vi "SP Append Measured Waveform.vi"(0 "Waveforms in":waveform(dbl)[](array[waveform]), 1 "Attribute Name (NI_ChannelName)":string="NI_ChannelName", 2 "CH Controls":T1[](array[typedef]) {"Measure" items=["S11", "S21", "S12", "S22"]; "Reference" format="%#.2g"; "Display Data" items=["Data", "Memory", "Data/Memory"]; "Format" items=["Log Mag", "Phase", "Expanded Phase", "Delay", "Smith", "Polar", "Lin Mag", "SWR", "Loss", "Real", "Imaginary"]; "Scale" min=0.001 step=1.0 format="%#.2g"; "Position" min=0.0 max=10.0}, 5 "Measured Data":cdb[](array[numeric]), 7 "All Measured Data":cdb[][](array[numeric]), 9 "Current Index":i32, 11 "error in (no error)":errorcluster, 12 "Number of Parameters Measured":i32, 14 "Measured Parameter":T4={"Stimulus Port"=1, "Response Port"=1} {"Stimulus Port" min=1 step=1; "Response Port" min=1 step=1}) -> (4 "Waveforms out":waveform(dbl)[](array[waveform]), 6 "Memory Exists?":bool, 10 "Stored Data":cdb[](array[numeric]), 15 "error out":errorcluster)   [LabVIEW 2011]
uses:
  TypeDefs/SP Parameter.ctl
  TypeDefs/SP Display Trace Controls.ctl
  TypeDefs/SP Display Format.ctl
  TypeDefs/SP Display Data.ctl
  TypeDefs/SP Format.ctl
  TypeDefs/SP Channel Type.ctl
panel:
  # "Div"
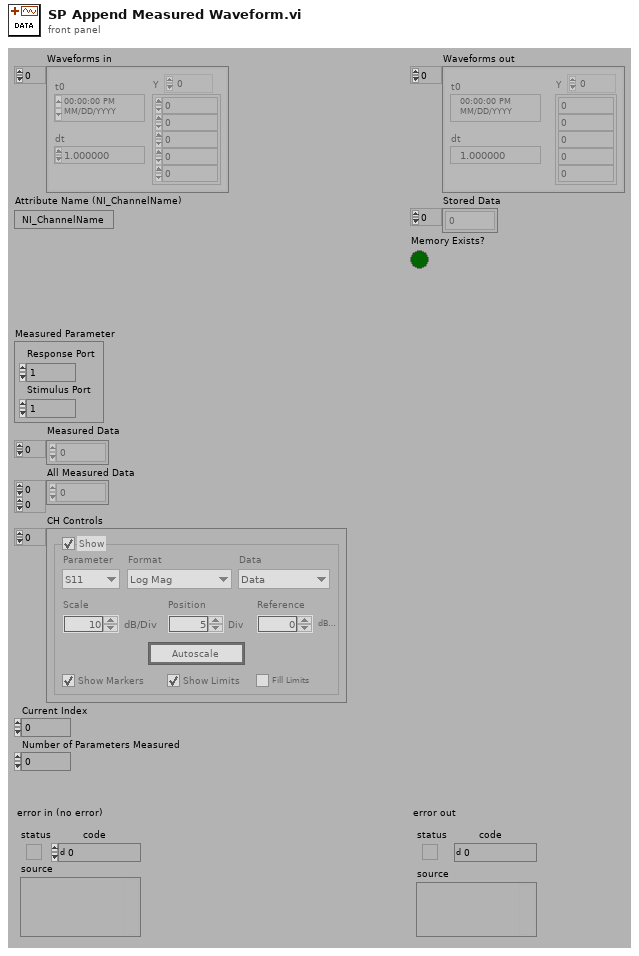
[diagram p1: front panel]
types:
  T1 = typedef "SP Display Trace Controls.ctl" = cluster{"Trace On":bool, "Measure":i32, "Format":T2, "Autoscale":bool, "Reference":dbl, "\nRefUnit":string, "Position":dbl, "Scale":dbl, "ScaleUnit":string, "LimitOn":bool, "LimitFill":bool, "Display Data":T3, "Show Markers":bool, "SXX":string}
  T2 = typedef "SP Display Format.ctl" = i32
  T3 = typedef "SP Display Data.ctl" = u16
  T4 = typedef "SP Parameter.ctl" = cluster{"Stimulus Port":i8, "Response Port":i8}
  T5 = typedef "SP Channel Type.ctl" = enum16{"Frequency", "Data", "Limit", "Adapter", "Memory", "Value", "Value Limit"}
  T6 = typedef "SP Format.ctl" = enum16{"Log Mag", "Lin Mag", "SWR", "Phase", "Expanded Phase", "Delay", "Insertion Loss", "Isolation", "Return Loss"}
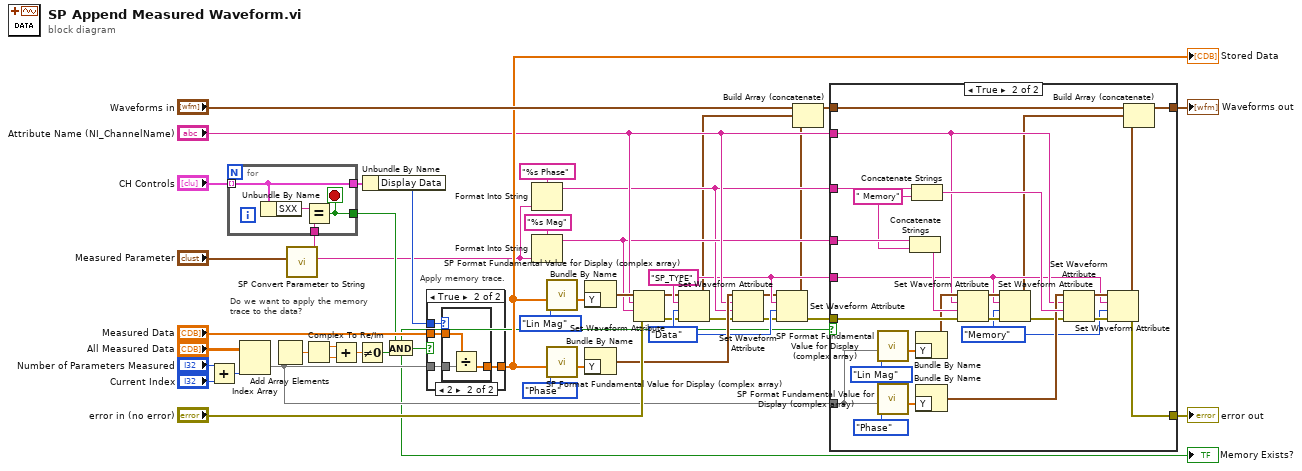
[diagram p0: block diagram]
diagram:
  w10 = "SP_TYPE" ("string")
  w11 = SP_Channel_Type."Data" ("Channel Type")
  # "Apply memory trace."
  # "Do we want to apply the memory\ntrace to the data?"
  n1 = Add(x="Number of Parameters Measured", y="Current Index") -> (x+y=w28:i32)
  n2 = Index Array(array="All Measured Data", index (col)=w28) -> (element=w14:cdb[])  [unwired: 1 in]
  n3 = Add Array Elements(numeric array=w14) -> (sum=w26:cdb)
  n4 = call "SP Convert Parameter to String.vi"("Parameter"="Measured Parameter") -> ("Parameter String"=w12:string)  [unwired: 10 out]
  n5 = for {
    tunnel: "CH Controls" -> [w48] mode=indexing
    tunnel: w12 -> [w49]
    tunnel: [w47] -> w21
    tunnel: [w48] -> w41
    stop <- w47 stop-if-true
    n6 = Unbundle By Name(w48) -> ("SXX"=w46:string)
    n7 = Equal?(x=w46, y=w49) -> (x = y?=w47:bool)
  }
  n8 = Complex To Re/Im(x + iy=w26) -> (x=w25:dbl, y=w24:dbl)
  n9 = Add(x=w25, y=w24) -> (x+y=w23:dbl)
  n10 = Not Equal To 0?(x=w23) -> (x != 0?=w1:bool)
  "Memory Exists?" <- w1
  n11 = Unbundle By Name(w41) -> ("Display Data"=w22:T3)
  n12 = And(x=w21, y=w1) -> (x .and. y?=w27:bool)
  n13 = case shown="True" w27 {
    tunnel: "Measured Data" -> [w50 w54]
    tunnel: [w50 w53] -> w29
    tunnel: w14 -> [_ w52]
    tunnel: w22 -> [_ w51]
    frame False {
    }
    frame True {
      n14 = case shown="2" w51 {
        tunnel: w54 -> [w55 w58]
        tunnel: [w55 w57] -> w53
        tunnel: w52 -> [_ w56]
        frame Default {
        }
        frame 2 {
          n15 = Divide(x=w58, y=w56) -> (x/y=w57:cdb[])
        }
      }
    }
  }
  "Stored Data" <- w29
  n16 = Format Into String(format string="%s Phase", w12) -> (resulting string=w17:string)  [unwired: 2 in, 1 out]
  n17 = Format Into String(format string="%s Mag", w12) -> (resulting string=w18:string)  [unwired: 2 in, 1 out]
  n18 = call "SP Format Fundamental Value for Display (complex array).vi"("Sxx Measured Format"=SP_Format."Lin Mag" ("Sxx Measure Format"), "Fundamental Values"=w29) -> ("Formatted Values"=w33:dbl[])  [unwired: 1 in, 8 out]
  n19 = call "SP Format Fundamental Value for Display (complex array).vi"("Sxx Measured Format"=SP_Format."Phase" ("Sxx Measure Format"), "Fundamental Values"=w29) -> ("Formatted Values"=w32:dbl[])  [unwired: 1 in, 8 out]
  n20 = Bundle By Name("Y"=w33) -> (w37:waveform(dbl))  [unwired: 1 out]
  n21 = Bundle By Name("Y"=w32) -> (w34:waveform(dbl))  [unwired: 1 out]
  n22 = Set Waveform Attribute(4:"error in (no error)", 5:w18, 6:"Attribute Name (NI_ChannelName)", 7:w37) -> (0:w4:errorcluster, 3:w5:waveform(dbl))  [unwired: 1 out]
  n23 = Set Waveform Attribute(4:w4, 5:w11, 6:w10, 7:w5) -> (0:w8:errorcluster, 3:w7:waveform(dbl))  [unwired: 1 out]
  n24 = Set Waveform Attribute(4:w8, 5:w17, 6:"Attribute Name (NI_ChannelName)", 7:w34) -> (0:w2:errorcluster, 3:w3:waveform(dbl))  [unwired: 1 out]
  n25 = Set Waveform Attribute(4:w2, 5:w11, 6:w10, 7:w3) -> (0:w9:errorcluster, 3:w6:waveform(dbl))  [unwired: 1 out]
  n26 = Build Array (concatenate)("Waveforms in", w7, w6) -> (w16:waveform(dbl)[])
  n27 = case shown="True" w1 {
    tunnel: w9 -> [w59 w86]
    tunnel: [w59 w63] -> w20
    tunnel: "Attribute Name (NI_ChannelName)" -> [_ w74]
    tunnel: w18 -> [_ w73]
    tunnel: w17 -> [_ w71]
    tunnel: w16 -> [w60 w83]
    tunnel: [w60 w82] -> w15
    tunnel: w14 -> [_ w77]
    tunnel: w10 -> [_ w65]
    frame False {
    }
    frame True {
      w66 = SP_Channel_Type."Memory" ("Channel Type")
      w72 = " Memory" ("string")
      n28 = call "SP Format Fundamental Value for Display (complex array).vi"("Sxx Measured Format"=SP_Format."Lin Mag" ("Sxx Measure Format"), "Fundamental Values"=w77) -> ("Formatted Values"=w80:dbl[])  [unwired: 1 in, 8 out]
      n29 = call "SP Format Fundamental Value for Display (complex array).vi"("Sxx Measured Format"=SP_Format."Phase" ("Sxx Measure Format"), "Fundamental Values"=w77) -> ("Formatted Values"=w81:dbl[])  [unwired: 1 in, 8 out]
      n30 = Concatenate Strings(w73, w72) -> (w85:string)
      n31 = Concatenate Strings(w71, w72) -> (w84:string)
      n32 = Bundle By Name("Y"=w80) -> (w76:waveform(dbl))  [unwired: 1 out]
      n33 = Bundle By Name("Y"=w81) -> (w75:waveform(dbl))  [unwired: 1 out]
      n34 = Set Waveform Attribute(4:w86, 5:w85, 6:w74, 7:w76) -> (0:w69:errorcluster, 3:w70:waveform(dbl))  [unwired: 1 out]
      n35 = Set Waveform Attribute(4:w69, 5:w66, 6:w65, 7:w70) -> (0:w64:errorcluster, 3:w61:waveform(dbl))  [unwired: 1 out]
      n36 = Set Waveform Attribute(4:w64, 5:w84, 6:w74, 7:w75) -> (0:w67:errorcluster, 3:w68:waveform(dbl))  [unwired: 1 out]
      n37 = Set Waveform Attribute(4:w67, 5:w66, 6:w65, 7:w68) -> (0:w63:errorcluster, 3:w62:waveform(dbl))  [unwired: 1 out]
      n38 = Build Array (concatenate)(w83, w61, w62) -> (w82:waveform(dbl)[])
    }
  }
  "Waveforms out" <- w15
  "error out" <- w20
